vi "GetTextPoint.vi"(10 "End Point":cluster{"X":i32, "Y":i32}, 11 "Y Offset":i32) -> (3 "Text Point":cluster{"X":i32, "Y":i32})   [LabVIEW 2024]
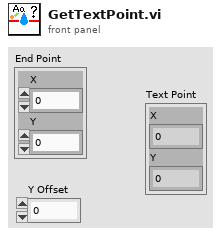
[diagram p1: front panel]
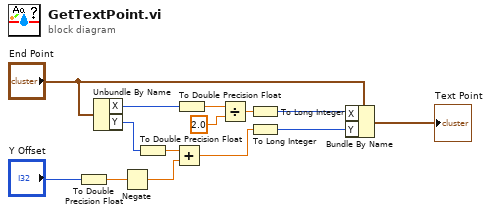
[diagram p0: block diagram]
diagram:
  n1 = To Double Precision Float(number="Y Offset") -> (double precision float=w2:dbl)
  n2 = Unbundle By Name("End Point") -> ("X"=w6:i32, "Y"=w11:i32)
  n3 = Negate(x=w2) -> (-x=w1:dbl)
  n4 = To Double Precision Float(number=w11) -> (double precision float=w12:dbl)
  n5 = Add(x=w12, y=w1) -> (x+y=w14:dbl)
  n6 = To Double Precision Float(number=w6) -> (double precision float=w7:dbl)
  n7 = Divide(x=w7, y=2.0) -> (x/y=w9:dbl)
  n8 = To Long Integer(number=w9) -> (32bit integer=w10:i32)
  n9 = To Long Integer(number=w14) -> (32bit integer=w13:i32)
  n10 = Bundle By Name(cluster="End Point", "X"=w10, "Y"=w13) -> (→"Text Point":cluster{"X":i32, "Y":i32})
